vi "Configure Language.vi"(0 "VISA resource name":refnum<visa-resource-name>, 5 "Language (0: Japanese)":u16(ring) items=["Japanese", "English", "German", "French", "Chinese", "Russian", "Korean"], 7 "Decimal Point Type (0: Point)":u16(ring) items=["Point", "Comma"], 11 "error in (no error)":errorcluster) -> (4 "VISA resource name out":refnum<visa-resource-name>, 15 "error out":errorcluster)   [LabVIEW 2020, in "Yokogawa GX Series.lvlib"]
doc: "Sets the language and decimal point type.\n\nCommands: SLang and SDPoint"
uses:
  <instrlib>/Yokogawa GX Series/Yokogawa GX Series.lvlib
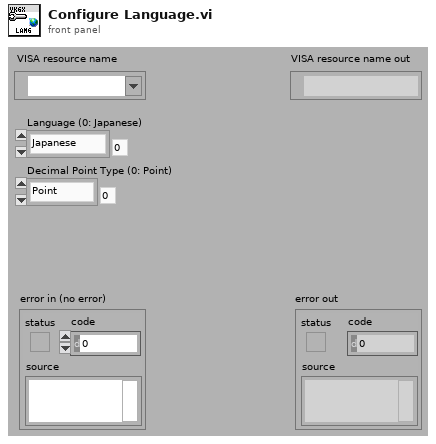
[diagram p1: front panel]
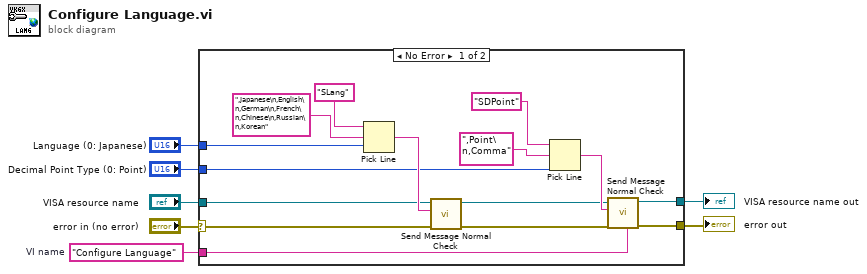
[diagram p0: block diagram]
diagram:
  w7 = "Configure Language"  # VI name
  n1 = case shown="No Error" "error in (no error)" {
    selector: "error in (no error)" -> [w8 w23]
    tunnel: w7 -> [w22 _]
    tunnel: [w21 w24] -> w6
    tunnel: "Language (0: Japanese)" -> [w18 _]
    tunnel: "VISA resource name" -> [w16 w24]
    tunnel: "Decimal Point Type (0: Point)" -> [w13 _]
    tunnel: [w11 w23] -> w2
    frame No Error {
      n2 = Pick Line(string ("")="SLang", multi-line string=",Japanese\n,English\n,German\n,French\n,Chinese\n,Russian\n,Korean", line index=w18) -> (output string=w17:string)
      n3 = call <instrlib>:"Send Message Normal Check.vi"("error in (no error)"=w8, "Send Message (\"\")"=w17, "VISA resource name"=w16) -> ("error out"=w9:errorcluster, "VISA resource name out"=w10:refnum<visa-resource-name>)  [unwired: 3 in, 4 out]
      n4 = Pick Line(string ("")="SDPoint", multi-line string=",Point\n,Comma", line index=w13) -> (output string=w12:string)
      n5 = call <instrlib>:"Send Message Normal Check.vi"("Source (\"\")"=w22, "error in (no error)"=w9, "Send Message (\"\")"=w12, "VISA resource name"=w10) -> ("error out"=w11:errorcluster, "VISA resource name out"=w21:refnum<visa-resource-name>)  [unwired: 2 in, 4 out]
    }
    frame Error {
    }
  }
  "error out" <- w2
  "VISA resource name out" <- w6
